vi "Error Test Label Count.vi"(6 "error text in":string, 8 "error in":errorcluster, 11 "array of elements":refnum<k20>[](array[refnum])) -> (0 "error out":errorcluster, 3 "array of elements out":refnum<k20>[](array[refnum]))   [LabVIEW 2020, in "ARINC 429 Import.lvlib"]
uses:
  ARINC 429 Import.lvlib
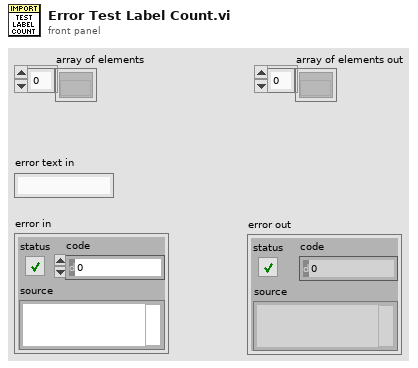
[diagram p1: front panel]
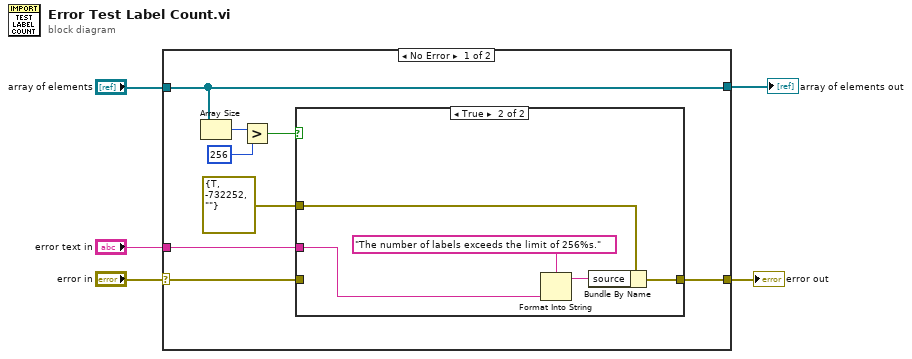
[diagram p0: block diagram]
diagram:
  n1 = case shown="No Error" "error in" {
    selector: "error in" -> [w11 w21]
    tunnel: [w13 w21] -> w4
    tunnel: [w10 w20] -> w3
    tunnel: "array of elements" -> [w10 w20]
    tunnel: "error text in" -> [w6 _]
    frame No Error {
      n2 = Array Size(array=w10) -> (size(s)=w9:i32)
      n3 = Greater?(x=w9, y=256) -> (0:w7:bool)
      n4 = case shown="True" w7 {
        tunnel: errorcluster {"status"=TRUE, "code"=-732252, "source"=""} ("error constant") -> [_ w18]
        tunnel: [w14 w19] -> w13
        tunnel: w11 -> [w14 _]
        tunnel: w6 -> [_ w15]
        frame False {
        }
        frame True {
          n5 = Format Into String(format string="The number of labels exceeds the limit of 256%s." ("source"), w15) -> (resulting string=w17:string)  [unwired: 2 in, 1 out]
          n6 = Bundle By Name(cluster=w18, "source"=w17) -> (w19:errorcluster)
        }
      }
    }
    frame Error {
    }
  }
  "error out" <- w4
  "array of elements out" <- w3
